vi "ST_parse_start_operation_response_pinion.vi"(6 "recordset_in":variant[][](array[variant]), 7 "Part exists?":bool, 8 "error_in":errorcluster, 11 "command_nmb":u8) -> (0 "error_out":errorcluster, 1 "user_ID":string, 2 "save_operation_to_SQL":bool, 3 "reference_data_to_PLC":u8[](array[numeric]))   [LabVIEW 2020]
uses:
  <vilib>/addons/database/_DB Variant To Data/Database Variant To Data.xnode
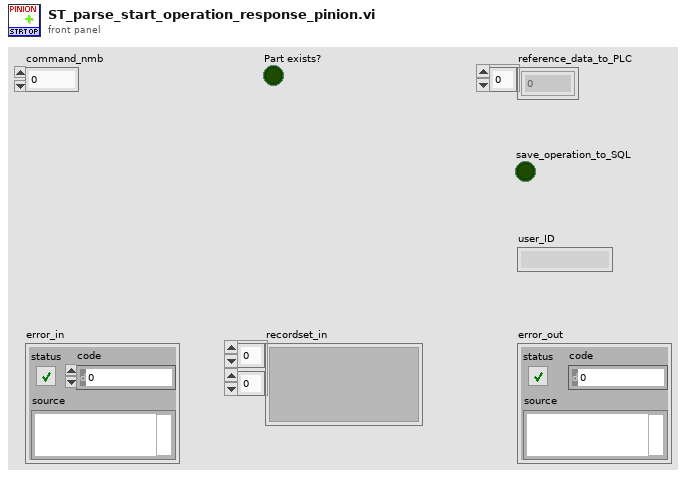
[diagram p1: front panel]
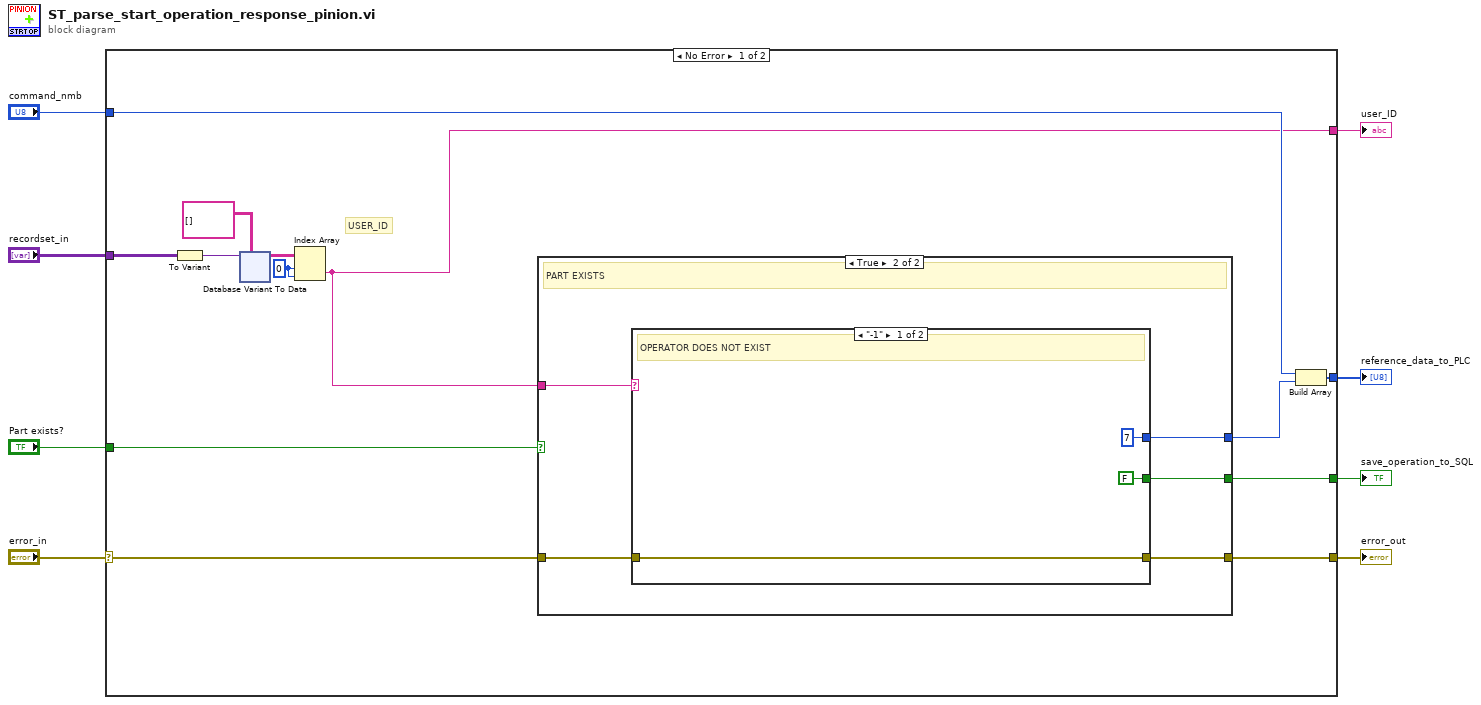
[diagram p0: block diagram]
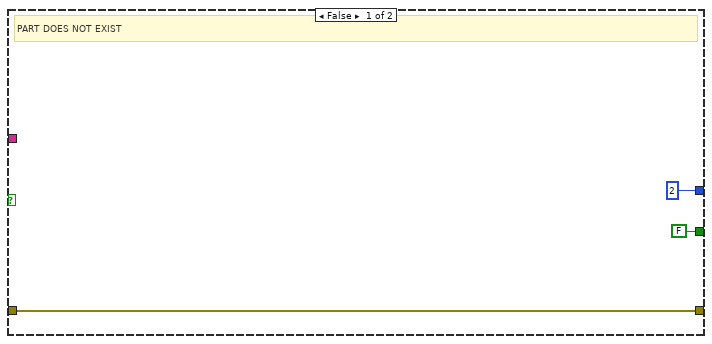
[diagram p2: hidden frame]
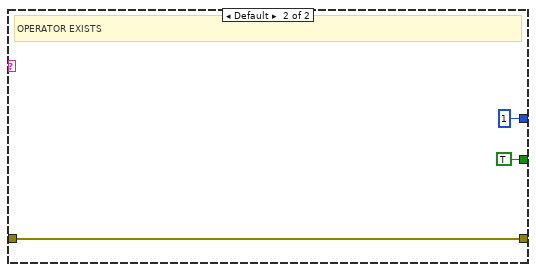
[diagram p3: hidden frame]
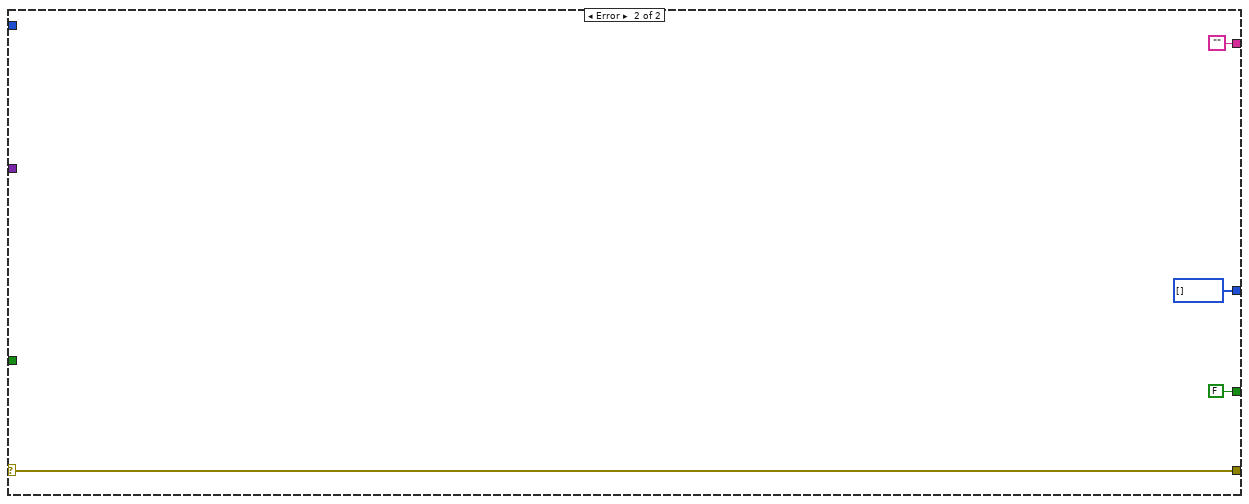
[diagram p4: hidden frame]
diagram:
  n1 = case shown="No Error" "error_in" {
    selector: "error_in" -> [w15 w71]
    tunnel: [w21 u8[] []] -> w3
    tunnel: "command_nmb" -> [w20 _]
    tunnel: "recordset_in" -> [w18 _]
    tunnel: [w14 w71] -> w5
    tunnel: [w12 FALSE] -> w4
    tunnel: [w9 ""] -> w2
    tunnel: "Part exists?" -> [w11 _]
    frame No Error {
      w10 = 0 ("index (row)")
      # "USER_ID"
      n2 = To Variant(anything=w18) -> (Variant=w17:variant)
      n3 = xnode "Database Variant To Data"("database variant"=w17, "type"=string[][] []) -> ("data"=w16:string[][])  [unwired: 1 in, 1 out]
      n4 = Index Array(array=w16, index (row)=w10, index (col)=w10) -> (element=w9:string)
      n5 = case shown="True" w11 {
        tunnel: [u8 2 w61] -> w13
        tunnel: w15 -> [w55 w60]
        tunnel: [w55 w59] -> w14
        tunnel: [FALSE w58] -> w12
        tunnel: w9 -> [_ w57]
        frame False {
          # "PART DOES NOT EXIST"
        }
        frame True {
          # "PART EXISTS"
          n6 = case shown="\"-1\"" w57 {
            tunnel: [u8 7 u8 1] -> w61
            tunnel: [FALSE TRUE] -> w58
            tunnel: w60 -> [w64 w65]
            tunnel: [w64 w65] -> w59
            frame "-1" {
              # "OPERATOR DOES NOT EXIST"
            }
            frame Default {
              # "OPERATOR EXISTS"
            }
          }
        }
      }
      n7 = Build Array(w20, w13) -> (w21:u8[])
    }
    frame Error {
    }
  }
  "error_out" <- w5
  "reference_data_to_PLC" <- w3
  "save_operation_to_SQL" <- w4
  "user_ID" <- w2
